vi "Topic Actor Core.vi"(8 "error in (no error)":errorcluster, 11 "Topic Actor in":refnum<class "Topic Actor.lvclass">) -> (0 "error out":errorcluster, 3 "Topic Actor out":refnum<class "Topic Actor.lvclass">)   [LabVIEW 2016, in "Stream Mediator.lvlib" / "Topic Actor.lvclass"]
doc: "--\nCopyright © 2017 Composed SystemsI All rights reserved.\n\nAuthor: Jon McBee <jon.mcbee@composed.io>\n\nThis library is provided \"AS IS\" ,WITHOUT WARRANTIES OR\nCONDITIONS OF ANY KIND, either express or implied.\n\nComposed Systems -- composed.io\n\nStream 0.0.1.1\nJon McBee - Composed Systems\nCopyright (c) 2017, Composed Systems"
uses:
  <userlib>/Composed Systems/Stream/Mediator/Classes/Topic Actor/Topic Actor.lvclass
  <userlib>/Composed Systems/Stream/Mediator/Classes/Topic Actor/Topic Actor.lvclass/Topic Actor.ctl
  <userlib>/Composed Systems/Stream/Mediator/Classes/Message Transport Queue/Message Transport Queue.lvclass
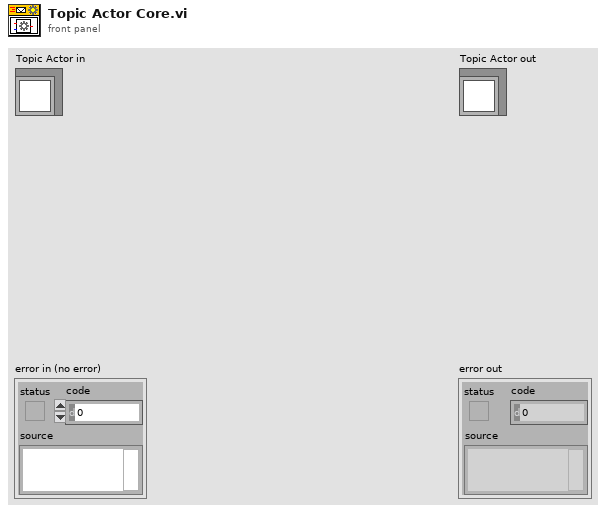
[diagram p1: front panel]
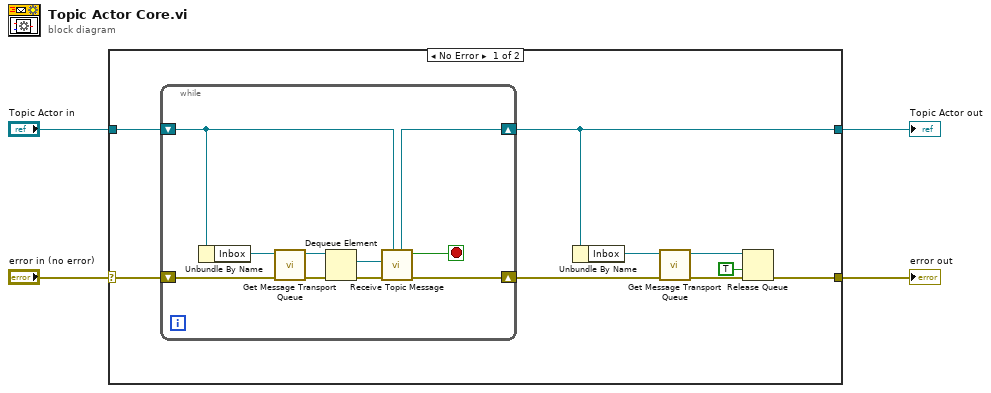
[diagram p0: block diagram]
diagram:
  n1 = case shown="No Error" "error in (no error)" {
    selector: "error in (no error)" -> [w12 w25]
    tunnel: [w10 w25] -> w3
    tunnel: [w11 w24] -> w2
    tunnel: "Topic Actor in" -> [w13 w24]
    frame No Error {
      n2 = while {
        shift-right: [w18] -> w11
        shift-left: w13 -> [w19]
        shift-right: [w16] -> w9
        shift-left: w12 -> [w23]
        stop <- w14 stop-if-true
        n3 = Unbundle By Name(w19) -> ("Inbox"=w22:refnum<class "Message Transport Queue.lvclass">)
        n4 = call <userlib>:"Get Message Transport Queue.vi"("error in (no error)"=w23, "Message Transport Queue in"=w22) -> ("error out"=w21:errorcluster, "Queue"=w20:refnum<queue>)  [unwired: 8 in]
        n5 = Dequeue Element(queue=w20, error in (no error)=w21) -> (element=w15:refnum<class "Message Interface.lvclass">, error out=w17:errorcluster)  [unwired: 1 in, 2 out]
        n6 = call-dynamic "Receive Topic Message.vi"("Topic Actor in"=w19, "error in (no error)"=w17, "Message in"=w15) -> ("error out"=w16:errorcluster, "Stop?"=w14:bool, "Topic Actor out"=w18:refnum<class "Topic Actor.lvclass">)  [unwired: 6 in]
      }
      n7 = Unbundle By Name(w11) -> ("Inbox"=w7:refnum<class "Message Transport Queue.lvclass">)
      n8 = call <userlib>:"Get Message Transport Queue.vi"("error in (no error)"=w9, "Message Transport Queue in"=w7) -> ("error out"=w8:errorcluster, "Queue"=w6:refnum<queue>)  [unwired: 8 in]
      n9 = Release Queue(queue=w6, force destroy? (F)=TRUE, error in (no error)=w8) -> (error out=w10:errorcluster)  [unwired: 2 out]
    }
    frame Error {
    }
  }
  "error out" <- w3
  "Topic Actor out" <- w2
